vi "set control mode.vi"(8 "error in (no error)":errorcluster, 10 "Start/stop controlling field":bool, 11 "VISA session":refnum<visa-resource-name>) -> (0 "error out":errorcluster, 3 "dup VISA session":refnum<visa-resource-name>)   [LabVIEW 2017]
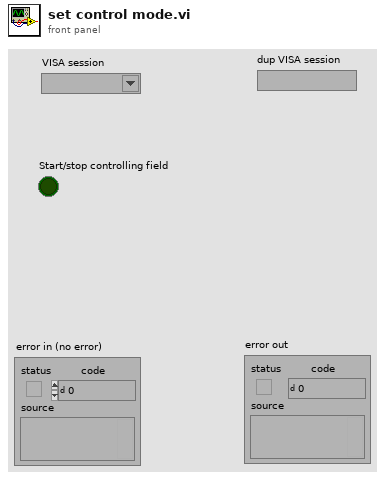
[diagram p1: front panel]
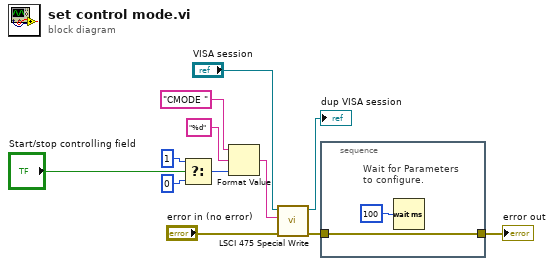
[diagram p0: block diagram]
diagram:
  n1 = Select(t=1, s="Start/stop controlling field", f=0) -> (s? t:f=w1:i32)
  n2 = Format Value(string ("")="CMODE ", format string="%d", value (0)=w1) -> (output string=w5:string)
  n3 = call "LSCI 475 Special Write.vi"("error in (no error)"="error in (no error)", "Write Buffer (\"\")"=w5, "VISA session"="VISA session") -> ("error out"=w7:errorcluster, "dup VISA session"=→"dup VISA session":refnum<visa-resource-name>)  [unwired: 6 in, 1 out]
  n4 = stacked-sequence {
    tunnel: w7 -> [w13]
    tunnel: [w13] -> w6
    frame #0 {
      # "Wait for Parameters\nto configure."
      n5 = Wait (ms)(milliseconds to wait=u32 100) -> ()  [unwired: 1 out]
    }
  }
  "error out" <- w6
